vi "Motor_Plus_Impedance_controller_monday24_G_compensation_2.vi"() -> ()   [LabVIEW 2016]
uses:
  <vilib>/Platform/TimedLoop/XDataNode/timing_clust.ctl
  <vilib>/Platform/TimedLoop/XDataNode/nitl_modes.ctl
  <vilib>/Platform/TimedLoop/XDataNode/wakeup.ctl
  <vilib>/Platform/TimedLoop/XDataNode/loadnilvce.vi
  <vilib>/Motion/Express/_s/nimc.ax.power.power.axis.vi
  <vilib>/Motion/Express/_s/nimc.fb.read.readExecutionData.axis.vi
  <vilib>/Motion/Express/_s/nimc.fb.straightLineMove.startStraightLineMove.axis.modeVelocity.0.vi
  <vilib>/Motion/Express/_s/nimc.fb.resetPosition.resetPosition.axis.vi
  <vilib>/Motion/Express/_s/nimc.fb.stopMove.stop.axis.modeDecelerate.vi
  <vilib>/Motion/Express/_s/nimc.ex.power.power.axis.vi
  <vilib>/platform/TimedLoop/XDataNode/XDataNode.xnode
  <vilib>/Motion/BlockNode/FB.NIMotion.xnode
  <vilib>/Platform/TimedLoop/XDataNode/XDNodeRunTimeDep.lvlib
panel:
  out "post sin 2":dbl format="%#_13g"
  out "motor torque, Nm 2":dbl format="%.3f"
  out "Torque 2":dbl(knob) scale=-1.0..2.0
  out "post sin":dbl format="%#_13g"
  out "pre sin":dbl format="%#_13g"
  in  "Position 2":dbl=0.25 format="%#_13g"
  out "Adjusted Motor Velocity":dbl format="%.3f"
  out "Adjusted Velocity":dbl(knob) scale=-1.0..2.0
  in  "Reset Position":bool
  in  "Position":dbl=0.25 format="%#_13g"
  in  "Speed":dbl=0.25 format="%#_12g"
  out "Torque":dbl(knob) scale=-3.0..3.0
  out "Position":dbl(knob) scale=-1.0..1.0
  out "Velocity":dbl(knob) scale=-1.0..5.0
  out "Load Cell":dbl(knob) scale=0.0..10.0
  in  "Move to Position?":bool
  out "Load cell, V":dbl format="%.3f"
  out "motor torque, Nm":dbl format="%.3f"
  out "motor velocity, rev/s":dbl format="%.3f"
  out "motor position, rev":dbl format="%.3f"
  in  "STOP VI":bool
  in  "Enable Axis \nControl":bool
  in  "Enable Motor \nDrive":bool
  in  "EMERGENCY MOTOR STOP":bool
  # "Raw Data from System"
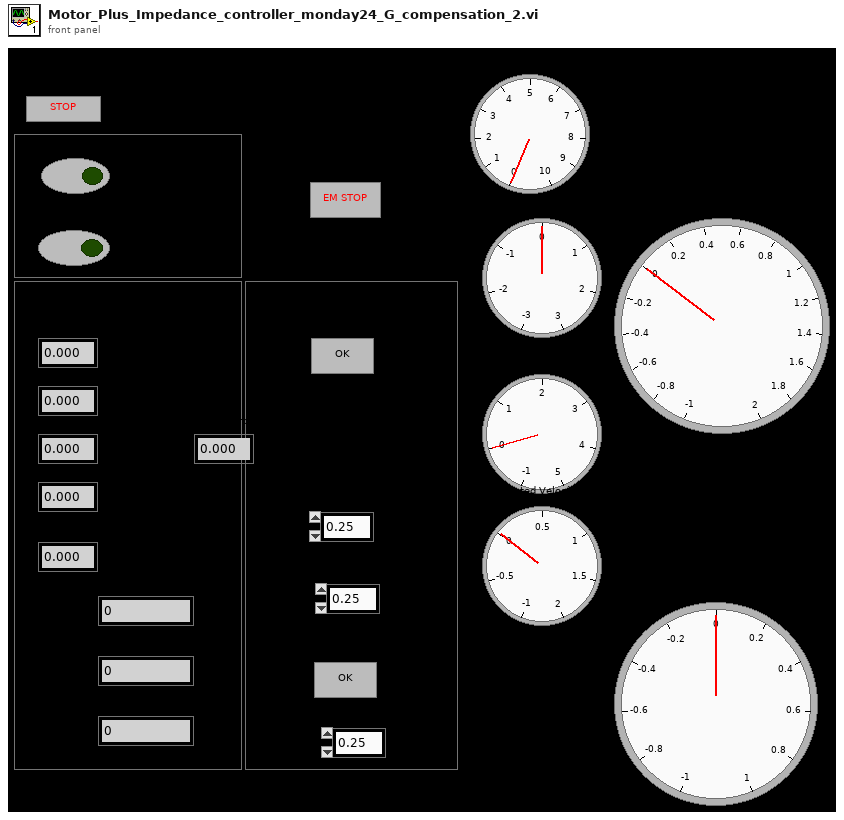
[diagram p1: front panel]
types:
  T1 = typedef "XDNodeRunTimeDep.lvlib/timing_clust.ctl" = cluster{"Expected End [f-1]":u64, "Actual End [f-1]":u64, "Finished Late? [f-1]":bool, "Expected End [i-1]":u64, "Actual End [i-1]":u64, "Finished Late? [i-1]":bool, "Expected Start [i]":u64, "Actual Start [i]":u64, "Expected Start [f]":u64, "Actual Start [f]":u64, "Source Name":string, "Structure Name":string, "Period":i64, "Deadline":i64, "Offset":i64, "Start":i64, "Priority":i32, "Timeout":i32, "Mode":T2, "Wakeup Reason":T3, "Error":errorcluster, "Source Type":string, "Secondary Source Type":string, "Global End Time":u64, "Global Start Time":u64, "Frame Duration":u64, "Iteration Duration":u64, "Assigned CPU":i32, "I/O Scan Engine Mode":u32}
  T2 = typedef "XDNodeRunTimeDep.lvlib/nitl_modes.ctl" = enum32{"No Change", "Process missed periods, maintain original phase", "Discard missed periods, maintain original phase", "Process missed periods, ignore original phase", "Discard missed periods, ignore original phase"}
  T3 = typedef "XDNodeRunTimeDep.lvlib/wakeup.ctl" = enum32{"Normal", "Aborted", "Asynchronous wakeup", "Timing source error", "Timed loop error", "Timeout"}
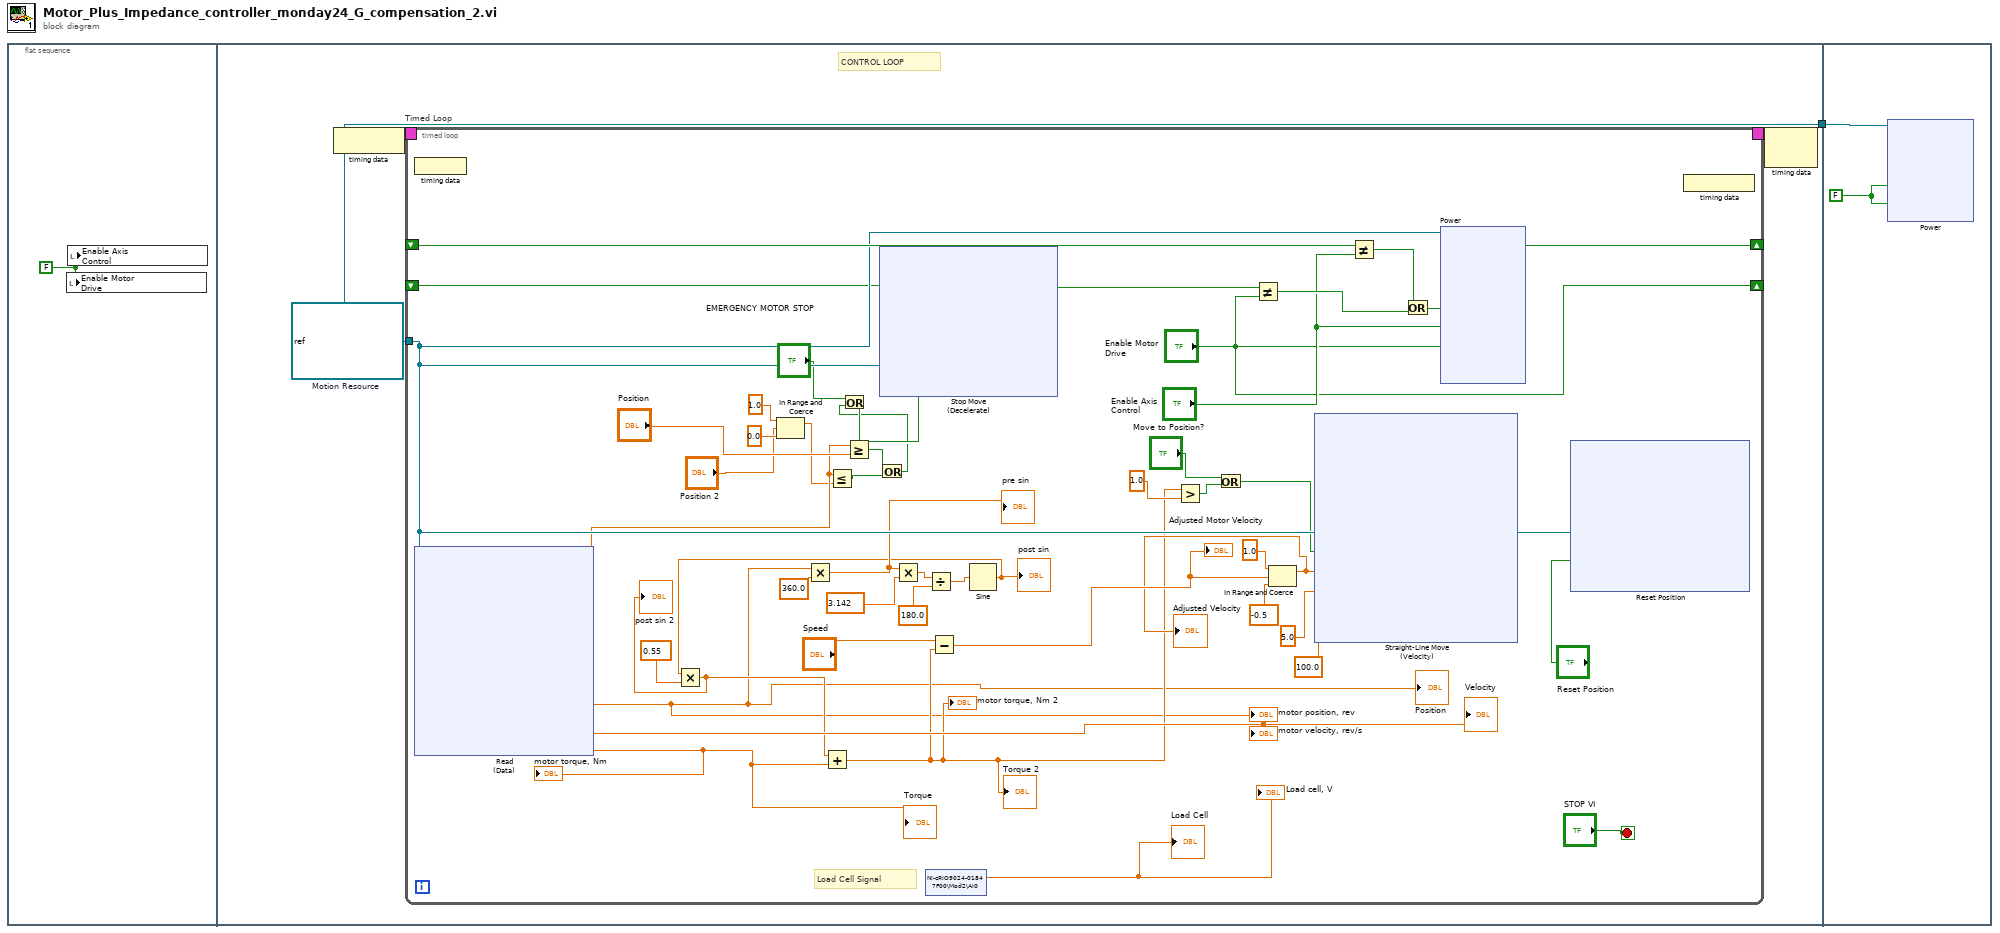
[diagram p0: block diagram]
diagram:
  n1 = flat-sequence {
    tunnel: [w5] -> w1
    tunnel: w1 -> [w129]
    frame #0 {
      w2 = FALSE
      n2 = local write "Enable Motor \nDrive"(w2) -> ()
      n3 = local write "Enable Axis \nControl"(w2) -> ()
    }
    frame #1 {
      w5 = refnum<k21> "nism://NI-cRIO9024-01847F00/Axis 1"  # Motion Resource
      # "CONTROL LOOP"
      n4 = node-c288() -> (w4:T1)
      n5 = timed-loop "Timed Loop" {
        tunnel: w5 -> [w43]
        timing: w4 -> [_]
        timing-out: [_] -> w3
        shift-right: ["Enable Axis \nControl"] -> _
        shift-left: _ -> [w50]
        shift-right: ["Enable Motor \nDrive"] -> _
        shift-left: _ -> [w35]
        stop <- "STOP VI" stop-if-true
        # "Load Cell Signal"
        n6 = node-c288() -> ()  [unwired: 1 in]
        n7 = xnode "Read\n(Data)"("resource"=w43) -> ("position"=w10:dbl, "torque"=w18:dbl, "velocity"=→"motor velocity, rev/s" →"Velocity":dbl)  [unwired: 1 in, 3 out]
        "motor position, rev" <- w10
        "motor torque, Nm" <- w18
        "Position" <- w10
        "Torque" <- w18
        n8 = In Range and Coerce(upper limit=1.0, x="Position 2", lower limit=0.0) -> (coerced(x)=w9:dbl)  [unwired: 1 out]
        n9 = Multiply(x=w10, y=360.0) -> (x*y=w33:dbl)
        "pre sin" <- w33
        n10 = Less Or Equal?(x=w10, y=w9) -> (x <= y?=w12:bool)
        n11 = Greater Or Equal?(x=w10, y="Position") -> (x >= y?=w13:bool)
        n12 = Or(x=w13, y=w12) -> (x .or. y?=w14:bool)
        n13 = Or(x="EMERGENCY MOTOR STOP", y=w14) -> (x .or. y?=w39:bool)
        n14 = xnode "Stop Move\n(Decelerate)"("resource"=w43, "execute"=w39) -> ()  [unwired: 1 in, 3 out]
        n15 = Multiply(x=w33, y=3.142) -> (x*y=w31:dbl)
        n16 = shared-variable "NI-cRIO9024-01847F00\\Mod2\\AI0"() -> (→"Load cell, V" →"Load Cell":dbl)  [unwired: 1 in, 1 out]
        n17 = Divide(x=w31, y=180.0) -> (x/y=w30:dbl)
        n18 = Sine(x=w30) -> (sin(x)=w19:dbl)
        "post sin" <- w19
        n19 = Multiply(x=w19, y=0.55) -> (x*y=w16:dbl)
        "post sin 2" <- w16
        n20 = Add(x=w16, y=w18) -> (x+y=w17:dbl)
        "Torque 2" <- w17
        "motor torque, Nm 2" <- w17
        n21 = Subtract(x="Speed", y=w17) -> (x-y=w26:dbl)
        "Adjusted Motor Velocity" <- w26
        n22 = Greater?(x=w17, y=1.0) -> (0:w22:bool)
        n23 = Or(x="Move to Position?", y=w22) -> (x .or. y?=w24:bool)
        n24 = Not Equal?(x=w35, y="Enable Motor \nDrive") -> (x != y?=w48:bool)
        n25 = In Range and Coerce(upper limit=1.0, x=w26, lower limit=-0.5) -> (coerced(x)=w25:dbl)  [unwired: 1 out]
        "Adjusted Velocity" <- w25
        n26 = xnode "Straight-Line Move\n(Velocity)"("resource"=w43, "execute"=w24, "velocity"=w25, "acceleration"=5.0, "deceleration"=100.0) -> ("resource out"=w40:refnum<k21>)  [unwired: 1 in, 2 out]
        n27 = Not Equal?(x=w50, y="Enable Axis \nControl") -> (x != y?=w49:bool)
        n28 = Or(x=w49, y=w48) -> (x .or. y?=w47:bool)
        n29 = xnode ("Power")("execute"=w47, "enable axis"="Enable Axis \nControl", "enable drive"="Enable Motor \nDrive", "resource"=w43) -> ()  [unwired: 1 in, 6 out]
        n30 = xnode "Reset Position"("resource"=w40, "execute"="Reset Position") -> ()  [unwired: 2 in, 3 out]
        n31 = node-c288() -> ()  [unwired: 1 out]
      }
      n32 = node-c288(w3) -> ()  [unwired: 1 out]
    }
    frame #2 {
      w130 = FALSE
      n33 = xnode ("Power")("enable axis"=w130, "enable drive"=w130, "resource"=w129) -> ()  [unwired: 1 in, 2 out]
    }
  }
